vi "Host Key Fingerprint.vi"(8 "Error In":errorcluster) -> (0 "Error Out":errorcluster)   [LabVIEW 2017, in "Tests.lvlib" / "Session.lvlib"]
uses:
  Session.lvlib
  src/LabSSH2/LabSSH2.lvlib
  src/LabSSH2/Public/SSH/Session.lvclass
  <vilib>/addons/_JKI Toolkits/Caraya/classes/Test/Test.lvclass
  <vilib>/addons/_JKI Toolkits/Caraya/classes/Assert/Assert.lvclass
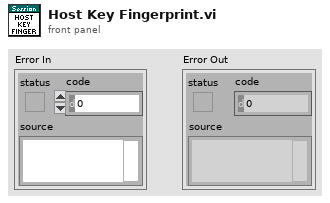
[diagram p1: front panel]
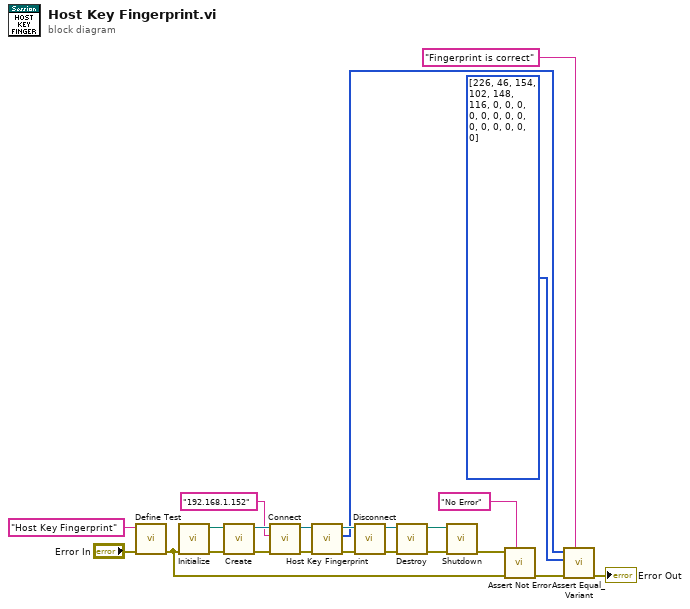
[diagram p0: block diagram]
diagram:
  n1 = call <vilib>:"Define Test.vi"("error in (no error)"="Error In", "Label (VI Title)"="Host Key Fingerprint") -> ("error out"=w18:errorcluster)  [unwired: 9 in]
  n2 = call "Initialize.vi"("Error In"=w18) -> ("Error Out"=w22:errorcluster, "labssh2 Shared Library Out"=w14:path)  [unwired: 9 in]
  n3 = call "Create.vi"("Error In"=w22, "labssh2 Shared Library"=w14) -> ("Error Out"=w12:errorcluster, "Sesssion"=w13:refnum<class "Session.lvclass">)  [unwired: 8 in]
  n4 = call "Connect.vi"("Error In"=w12, "Address"="192.168.1.152", "Session In"=w13) -> ("Error Out"=w5:errorcluster, "Sesssion Out"=w8:refnum<class "Session.lvclass">)  [unwired: 7 in]
  n5 = call "Host Key Fingerprint.vi"("Error In"=w5, "Session In"=w8) -> ("Error Out"=w6:errorcluster, "Fingerprint"=w3:u8[], "Sesssion Out"=w7:refnum<class "Session.lvclass">)  [unwired: 7 in]
  n6 = call "Disconnect.vi"("Error In"=w6, "Session In"=w7) -> ("Error Out"=w10:errorcluster, "Sesssion Out"=w11:refnum<class "Session.lvclass">)  [unwired: 8 in]
  n7 = call "Destroy.vi"("Error In"=w10, "Session"=w11) -> ("Error Out"=w20:errorcluster, "labssh2 Shared Library"=w21:path)  [unwired: 8 in]
  n8 = call "Shutdown.vi"("Error In"=w20, "labssh2 Shared Library"=w21) -> ("Error Out"=w19:errorcluster)  [unwired: 9 in]
  n9 = call <vilib>:"Assert Not Error.vi"("Label"="No Error", "error in (no error)"=w18, "Not Error?"=w19) -> ("error out"=w17:errorcluster)  [unwired: 8 in]
  n10 = call <vilib>:"Assert Equal_Variant.vi"("Label"="Fingerprint is correct", "error in (no error)"=w17, "Y"=u8[] [226, 46, 154, 102, 148, 116, 0, 0, 0, 0, 0, 0, 0, 0, 0, 0, 0, 0, 0, 0] ("Fingerprint"), "X"=w3) -> ("error out"=→"Error Out":errorcluster)  [unwired: 7 in]
